vi "initialize_driver_session.vi"(4 "Supported instruments":string[](array[string]), 5 "Repeated Capabilities":T4[](array[typedef]), 6 "Attributes":T2[](array[typedef]) {"Flags" format="%08b"; "Access" items=["Read Only", "Write Only", "Read/Write"]; "Data Type" items=["Integer 32", "Double", "String", "Boolean", "None", "Integer 64", "RawString"]}, 7 "Range Tables":T3[](array[typedef]) {"Type" items=["Range", "Coerced", "Discrete"]}, 8 "error in":errorcluster caption="error in (no error)", 9 "Option String":string, 10 "Non-VXI sessions list (\"ASRL,SOCKET\")":T1[](array[typedef])=[enum."ASRL", enum."SOCKET"], 11 "VISA resource name":refnum<visa-resource-name>) -> (0 "error out":errorcluster, 2 "Simulation *IDN? response out":string, 3 "VISA resource name out":refnum<visa-resource-name>)   [LabVIEW 2020, in "Rohde&Schwarz RTx Oscilloscopes.lvlib" / "rsidr_core.lvlib"]
uses:
  rsidr_core.lvlib
  type_Input_Format_RepCap.ctl
  type_Input_Format_RangeTable.ctl
  type_Input_Format_Attribute.ctl
  type_InterfaceType.ctl
  type_Error_Codes.ctl
  type_Session_Parameter_int32.ctl
  type_Session_Data.ctl
  type_VisaAccessMode.ctl
  type_OPC_Wait_Mode.ctl
  type_Binary_Float_Number_Format.ctl
  type_Binary_Integer_Number_Format.ctl
  _type_Operation_Fgv_Attributes.ctl
  _type_Operation_Fgv_Cache.ctl
  _type_Operation_Fgv_RangeTable.ctl
  type_AdditionalFlag_Bits.ctl
  _type_Operation_Fgv_Session.ctl
  type_Session_Parameter_Boolean.ctl
  Match Regular Expression.xnode
  _type_Operation_Fgv_Debug.ctl
panel:
  # "Attribute Flags:\nbit 0: OPC Wait\nbit 1: No Status Check\nbit 2: Cache only\nbit 3: Hidden"
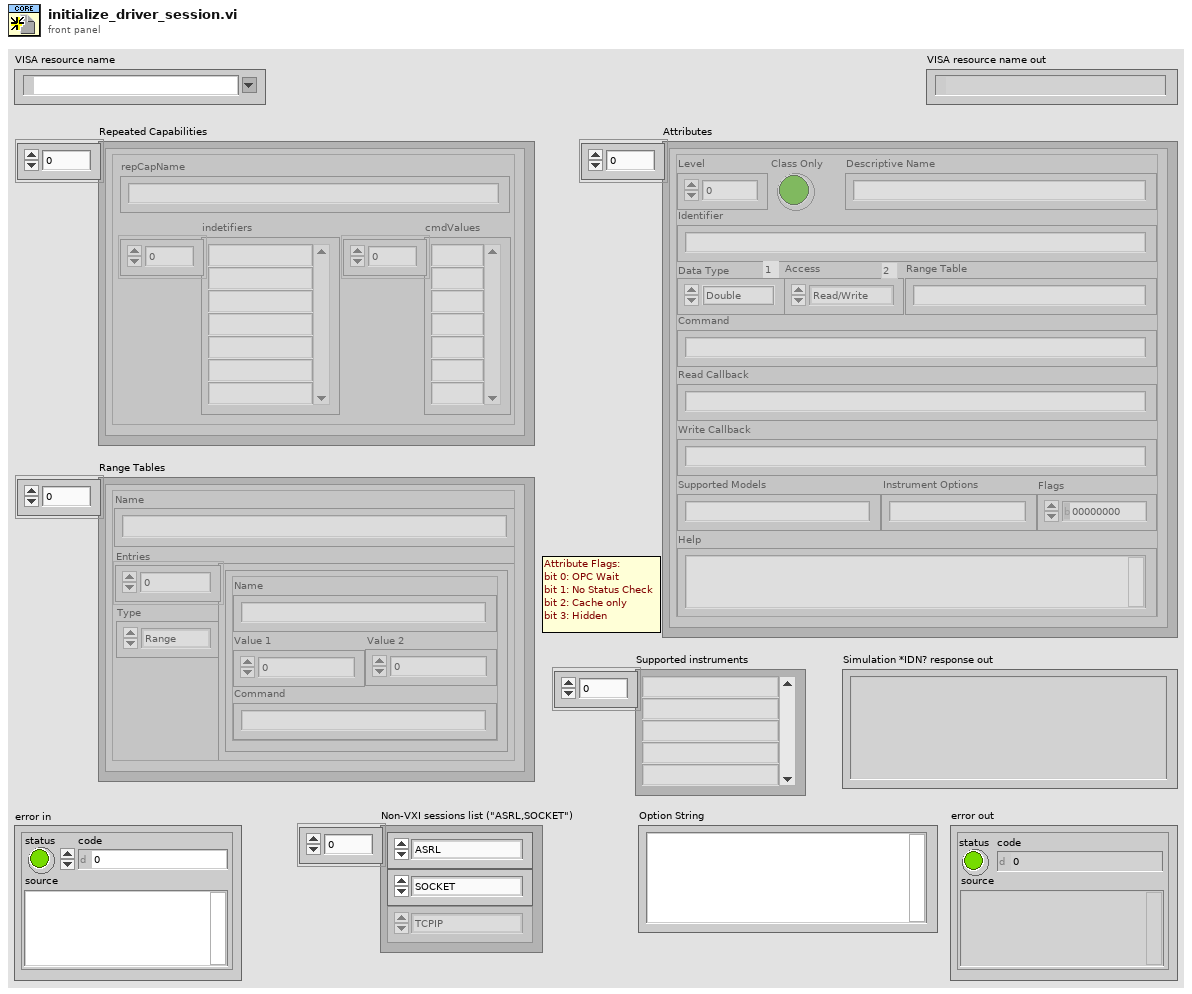
[diagram p1: front panel]
types:
  T1 = typedef "Rohde&Schwarz RTx Oscilloscopes.lvlib/rsidr_core.lvlib/type_InterfaceType.ctl" = enum16{"Unknown", "GPIB", "VXI", "GPIB_VXI", "ASRL", "PXI", "TCPIP", "USB", "SOCKET"}
  T2 = typedef "Rohde&Schwarz RTx Oscilloscopes.lvlib/rsidr_core.lvlib/type_Input_Format_Attribute.ctl" = cluster{"Level":i32, "Class Only":bool, "Identifier":string, "Descriptive Name":string, "Data Type":u16, "Command":string, "Access":u16, "Range Table":string, "Read Callback":string, "Write Callback":string, "Supported Models":string, "Instrument Options":string, "Flags":i32, "Help":string}
  T3 = typedef "Rohde&Schwarz RTx Oscilloscopes.lvlib/rsidr_core.lvlib/type_Input_Format_RangeTable.ctl" = cluster{"Type":u16, "Name":string, "Entries":cluster{"Name":string, "Value 1":dbl, "Value 2":dbl, "Command":string}[]}
  T4 = typedef "Rohde&Schwarz RTx Oscilloscopes.lvlib/rsidr_core.lvlib/type_Input_Format_RepCap.ctl" = cluster{"repCapName":string, "indetifiers":string[], "cmdValues":string[]}
  T5 = typedef "Rohde&Schwarz RTx Oscilloscopes.lvlib/rsidr_core.lvlib/_type_Operation_Fgv_RangeTable.ctl" = enum16{"Initialize", "Check", "Coerce", "Get Command String", "Get Numeric Value", "Get Default Value", "Get Range Table Type"}
  T6 = typedef "Rohde&Schwarz RTx Oscilloscopes.lvlib/rsidr_core.lvlib/_type_Operation_Fgv_Cache.ctl" = enum16{"Initialize", "Get Cached Value", "Set Cached Value", "Clear"}
  T7 = typedef "Rohde&Schwarz RTx Oscilloscopes.lvlib/rsidr_core.lvlib/_type_Operation_Fgv_Attributes.ctl" = enum16{"Initialize", "Get Attribute"}
  T8 = typedef "Rohde&Schwarz RTx Oscilloscopes.lvlib/rsidr_core.lvlib/type_Session_Data.ctl" = cluster{"IDN string":string, "Instrument FW":string, "Instr type":string, "Instr type for err. msg.":string, "Installed Options":string[], "Ignore Error Messages":string, "Logging params":variant, "OPC Timeout":i32, "VISA Timeout":i32, "STB Poll VISA Timeout":i32, "Additional Flags":i32, "Wait Before Read":i32, "Wait Before Write":i32, "Option String Flags":i32, "IO Segment Size":i64, "VISA Access Mode":T9, "Interface Type":T1, "OPC Wait Mode":T10, "Bin Float Number  Format":T11, "Bin Integer Number Format":T12, "Simulate":bool, "VXIcapable":bool, "Duplicate Session":bool, "Add LF to Write":bool, "Logging":bool, "Fast Sweep":bool, "Query Instrument Status":bool, "Check Range":bool, "Check Options":bool, "OPC-sync Attr Writes":bool, "OPC-sync Attr Queries":bool}
  T9 = typedef "Rohde&Schwarz RTx Oscilloscopes.lvlib/rsidr_core.lvlib/type_VisaAccessMode.ctl" = u16
  T10 = typedef "Rohde&Schwarz RTx Oscilloscopes.lvlib/rsidr_core.lvlib/type_OPC_Wait_Mode.ctl" = enum16{"STBpolling", "STBpollingSlow", "STBpollingSuperSlow", "ServiceRequest", "OPCquery"}
  T11 = typedef "Rohde&Schwarz RTx Oscilloscopes.lvlib/rsidr_core.lvlib/type_Binary_Float_Number_Format.ctl" = enum16{"Float_4_Bytes_Swapped", "Float_4_Bytes", "Double_8_Bytes_Swapped", "Double_8_Bytes"}
  T12 = typedef "Rohde&Schwarz RTx Oscilloscopes.lvlib/rsidr_core.lvlib/type_Binary_Integer_Number_Format.ctl" = enum16{"Int32_4_Bytes_Swapped", "Int32_4 Bytes", "Int16_2_Bytes_Swapped", "Int16_2_Bytes"}
  T13 = typedef "Rohde&Schwarz RTx Oscilloscopes.lvlib/rsidr_core.lvlib/type_Session_Parameter_int32.ctl" = enum16{"OPC Timeout", "Additional Flags", "Wait Before Write", "Wait Before Read", "Bin Data Chunk Size", "VISA Access Mode", "VISA Timeout", "Bin Float Number Format", "Bin Integer Number Format", "STBpollVISAtimeout", "OPCwaitMode"}
  T14 = typedef "Rohde&Schwarz RTx Oscilloscopes.lvlib/rsidr_core.lvlib/type_Error_Codes.ctl" = enum16{"No_error", "VISA_err_ResourceNotFound", "VISA_err_Timeout", "VISA_warn_MoreDataAvailable", "RS_err_MissingCallback", "RS_err_InvalidAttribute", "RS_err_InvalidValue", "RS_err_UnknownResource", "RS_err_AlreadyInitialized", "RS_err_InstrumentStatus", "RS_err_BadRepCapName", "RS_err_TypesMismatch", "RS_err_ValueNotSupported", "RS_err_InvalidRngTable", "RS_err_IDqueryFail", "RS_err_UnexpResponse", "VISA_warn_ConfigNotLoaded", "RS_err_AttributeNotReadable", "RS_err_AttributeNotWritable", "RS_err_InstrumentType", "RS_err_InstrumentOption", "VISA_err_InvalidSize", "RS_err_ReliabilityIndicator", "VISA_warn_UnknownStatus", "VISA_warn_TermCharRead", "VISA_err_IO_error", "RS_err_FunctionNotSupported", "VISA_warn_QueueEmpty"}
  T15 = typedef "Rohde&Schwarz RTx Oscilloscopes.lvlib/rsidr_core.lvlib/type_AdditionalFlag_Bits.ctl" = enum16{"Send LF after Bin Block", "Junk read with io_clear_buffers.vi", "io_clear_buffers: viClear()", "io_clear_buffers: viFlush()", "<NotUsed1>", "Allow Dbl & Int Bin/Ascii read", "*OPC? in check_instrument_error.vi", "<NotUsed2>", "Smart Enum Matching", "Less Strict RepCaps check", "AssureResponseEndWithLF"}
  T16 = typedef "Rohde&Schwarz RTx Oscilloscopes.lvlib/rsidr_core.lvlib/_type_Operation_Fgv_Session.ctl" = enum16{"Initialize", "GetData", "SetData", "Clear", "GetSessionIx"}
  T17 = typedef "Rohde&Schwarz RTx Oscilloscopes.lvlib/rsidr_core.lvlib/type_Session_Parameter_Boolean.ctl" = enum16{"Simulate", "Query Instr Status", "Check Range", "Check Options", "Add LF to Write", "Duplicate Session", "Fast Sweep", "Logging", "OPC-sync Attribute Queries", "OPC-sync Attribute Writes"}
  T18 = enum16{"Unknown", "GPIB", "VXI", "GPIB_VXI", "ASRL", "PXI", "TCPIP", "USB", "SOCKET"}
  T19 = typedef "Rohde&Schwarz RTx Oscilloscopes.lvlib/rsidr_core.lvlib/_type_Operation_Fgv_Debug.ctl" = enum16{"Reset", "ReadCommand", "SetCommand"}
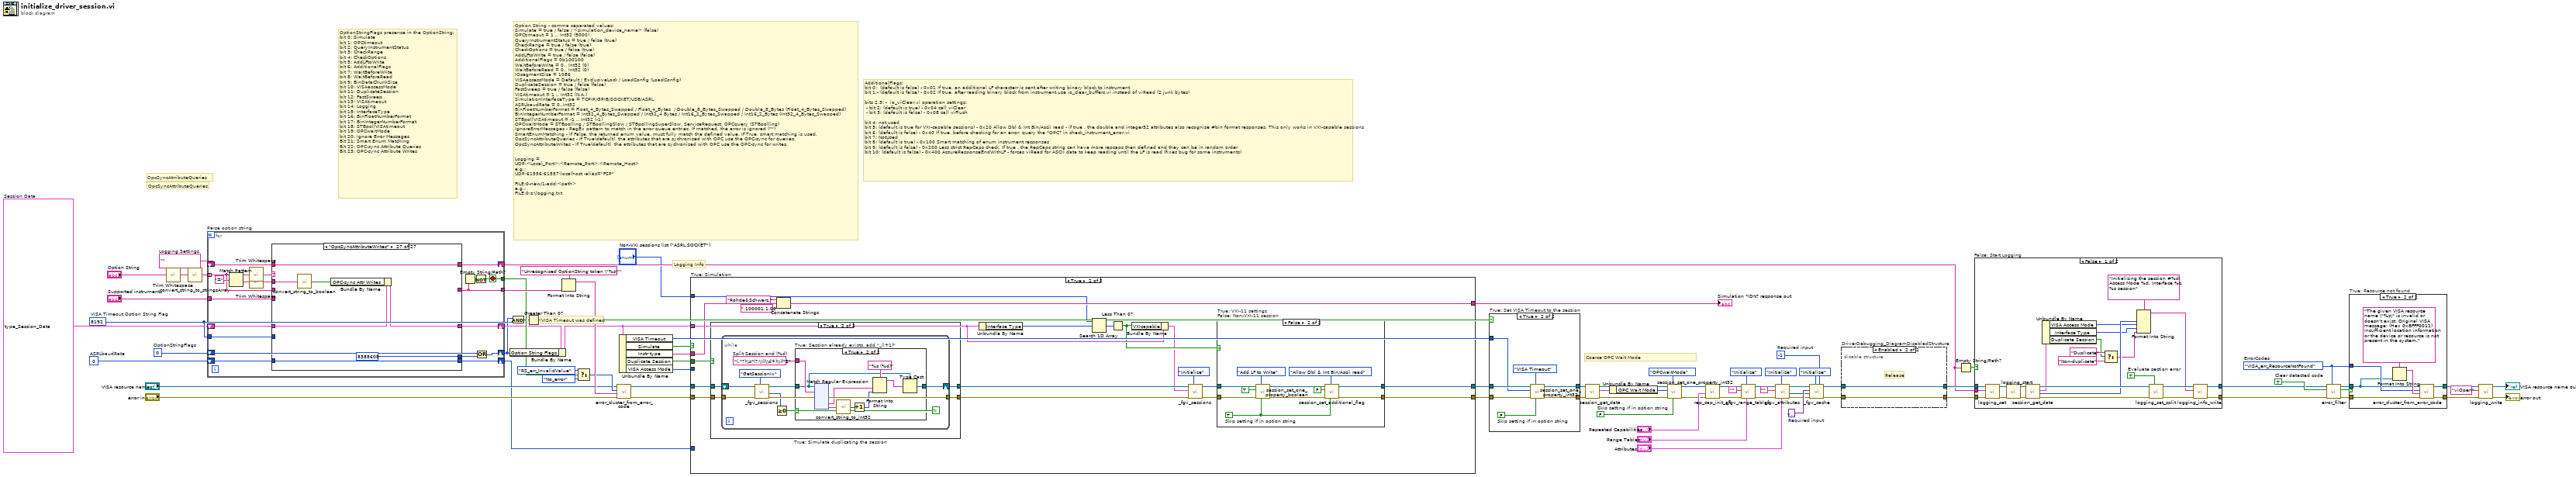
[diagram p0: block diagram]
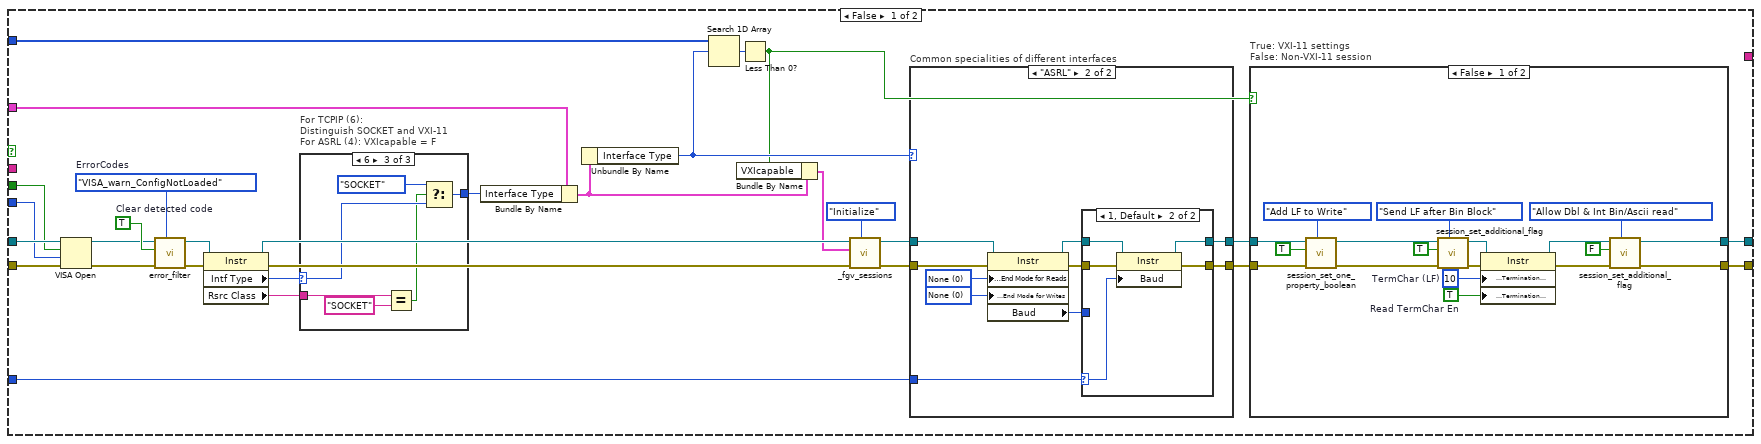
[diagram p3: hidden frame]
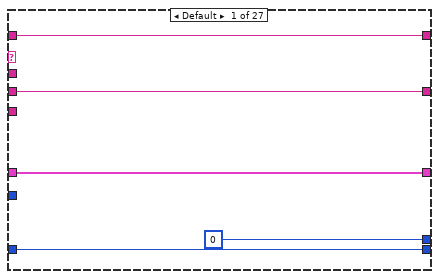
[diagram p14: hidden frame]
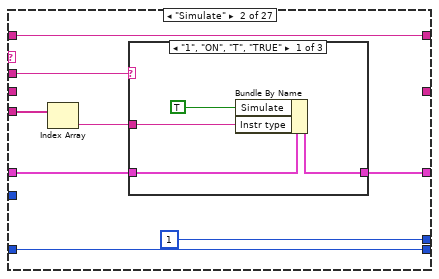
[diagram p15: hidden frame]
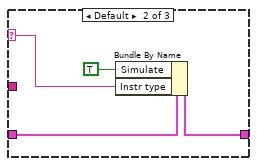
[diagram p16: hidden frame]
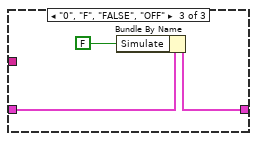
[diagram p17: hidden frame]
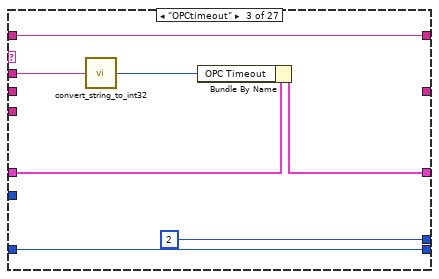
[diagram p18: hidden frame]
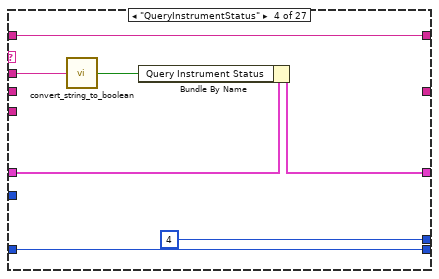
[diagram p19: hidden frame]
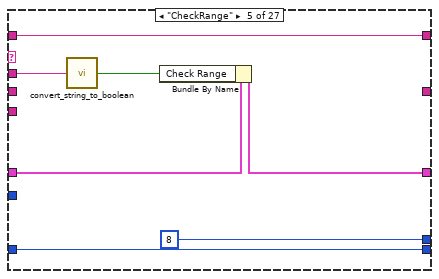
[diagram p20: hidden frame]
diagram:
  w4 = T8 {"IDN string"="", "Instrument FW"="", "Instr type"="", "Instr type for err. msg."="", "Installed Options"=[], "Ignore Error Messages"="", "Logging params"=variant, "OPC Timeout"=10000, "VISA Timeout"=5000, "STB Poll VISA Timeout"=-1, "Additional Flags"=292, "Wait Before Read"=0, "Wait Before Write"=0, "Option String Flags"=0, "IO Segment Size"=10000000, "VISA Access Mode"=4, "Interface Type"=enum."Unknown", "OPC Wait Mode"=enum."STBpolling", "Bin Float Number  Format"=enum."Float_4_Bytes_Swapped", "Bin Integer Number Format"=enum."Int32_4_Bytes_Swapped", "Simulate"=FALSE, "VXIcapable"=FALSE, "Duplicate Session"=FALSE, "Add LF to Write"=FALSE, "Logging"=FALSE, "Fast Sweep"=FALSE, "Query Instrument Status"=TRUE, "Check Range"=TRUE, "Check Options"=TRUE, "OPC-sync Attr Writes"=TRUE, "OPC-sync Attr Queries"=TRUE}  # Session Data
  w7 = FALSE  # Skip setting if in option string
  w18 = 0  # ASRLbaudRate
  w31 = 8192  # VISA Timeout Option String Flag
  w37 = 0  # OptionStringFlags
  w57 = type_Error_Codes."VISA_err_ResourceNotFound"  # ErrorCodes
  w59 = TRUE  # Clear detected code
  w66 = ""  # Logging Settings
  w80 = variant  # Required input
  w38 = -1  # Required input
  # "OpcSyncAttributeQueries"
  # "OpcSyncAtrributeQueries"
  # "Coerce OPC Wait Mode"
  # "VISA Timeout was defined"
  # "Logging Info"
  # "OptionStringFlags presence in the OptionString:\nbit 0: Simulate\nbit 1: OPCtimeout\nbit 2: QueryInstrumentStatus\nbit 3: CheckRange\nbit 4: CheckOptions\nbit 5: AddLFtoWrite\nbit 6: AdditionalFlags\nbit 7: WaitBeforeWrite\nbit 8: WaitBeforeRead\nbit 9: BinDataChunkSize\nbit 10: VISAaccessMode\nbit 11: DuplicateSession\nbit 12: FastSweep\nbit 13: VISAtimeout\nbit 14: Logging\nbit 15: InterfaceType\nbit 16: BinFloatNumberFormat\nbit 17: BinIntegerNumberFormat\nbit 18: STBpollVISAtimeout\nbit 19: OPCwaitMode\nbit 20: Ignore Error Messages\nBit 21: Smart Enum Matching\nBit 22: OPC-sync Attribute Queries\nBit 23: OPC-sync Attribute Writes"
  # "AdditionalFlags:\nbit 0:  (default is false) - 0x01 If true, an additional LF characterr is sent after writing binary block to instrument\nbit 1:- (default is false) - 0x02 If true, after reading binary block from instrument use io_clear_buffers.vi instead of viRead (2 junk bytes)\n\nbits 2,3: -  io_viClear.vi operation settings:\n - bit 2: (default is true) - 0x04 call viClear\n - bit 3: (default is false) - 0x08 call viFlush\n\nbit 4: not used\nbit 5: (default is true for VXI-capable sessions) - 0x20 Allow Dbl & Int Bin/Ascii read - if true , the double and integer32 attributes also recognise #bin format responses. This only works in VXI-capable sessions\nbit 6: (default is false) - 0x40 If true, before checking for an error, query the *OPC? in check_instrument_error.vi\nbit 7: NotUsed\nbit 8: (default is true) - 0x100 Smart matching of enum instrument responses\nbit 9: (default is false) - 0x200 Less strict RepCaps check. If true , the RepCaps string can have more repcaps then defined and they can be in random order\nbit 10: (default is false) - 0x400 AssureResponseEndWithLF - forces viRead for ASCII data to keep reading until the LF is read (fixes bug for some instruments)"
  # "Option String - comma separated values:\nSimulate = true / false / <simulation_device_name> (false)\nOPCtimeout = 1 .. Int32 (5000)\nQueryInstrumentStatus = true / false (true)\nCheckRange = true / false (true)\nCheckOptions = true / false (true)\nAddLFtoWrite = true / false (false)\nAdditionalFlags = 0b100100\nWaitBeforeWrite = 0.. Int32 (0)\nWaitBeforeRead = 0.. Int32 (0)\nIOsegmentSize = 10E6\nVISAaccessMode = Default / ExclusiveLock / LoadConfig (LoadConfig)\nDuplicateSession = true / false (false)\nFastSweep = true / false (false)\nVISAtimeout = 1 .. Int32 (N.A.)\nSimulationInterfaceType = TCPIP/GPIB/SOCKET/USB/ASRL\nASRLbaudRate = 0..Int32\nBinFloatNumberFormat = Float_4_Bytes_Swapped / Float_4_Bytes  / Double_8_Bytes_Swapped / Double_8_Bytes (Float_4_Bytes_Swapped)\nBinIntegerNumberFormat = Int32_4_Bytes_Swapped / Int32_4 Bytes / Int16_2_Bytes_Swapped / Int16_2_Bytes (Int32_4_Bytes_Swapped)\nSTBpollVISAtimeout = -1 .. Int32 (-1)\nOPCwaitMode = STBpolling / STBpollingSlow / STBpollingSuperSlow, ServiceRequest, OPCquery (STBpolling)\nIgnoreErrorMessages - RegEx pattern to match in the error queue entries. If matched, the error is ignored (\"\")\nSmartEnumMatching - If False, the returned enum value. must fully match the defined value. If True, smart matching is used.\nOpcSyncAttributeQueries - If True(default), the attributes that are sychronised with OPC use the OPC-sync for queries.\nOpcSyncAttributeWrites - If True(default), the attributes that are sychronised with OPC use the OPC-sync for writes.\n\n\nLogging =\nUDP:<Local_Port>:<Remote_Port>:<Remote_Host>\ne.g.:\nUDP:61556:61557:localhost -alias=\"FSP\"\n\nFILE:0-new/1-add:<path>\ne.g.:\nFILE:0:c:\\logging.txt"
  n1 = call "Trim Whitespace.vi"("string"="Option String") -> ("trimmed string"=w6:string)  [unwired: 1 in]
  n2 = call "convert_string_to_stringsArray.vi"("String in"=w6) -> ("string array out"=w70:string[])  [unwired: 3 in, 1 out]
  n3 = for "Parse option string" {
    tunnel: w70 -> [w94] mode=indexing
    shift-right: [w96] -> w33
    shift-left: w4 -> [w97]
    tunnel: "Supported instruments" -> [w92]
    shift-right: [w90] -> w64
    shift-left: w66 -> [w91]
    tunnel: [w88] -> w44
    tunnel: [w87] -> w43
    shift-right: [w85] -> w32
    shift-left: w37 -> [w86]
    tunnel: w31 -> [w83]
    shift-right: [w81] -> w17
    shift-left: w18 -> [w82]
    stop <- w87 stop-if-true
    n4 = Match Pattern(string=w94, regular expression="=") -> (before substring=w99:string, after substring=w98:string)  [unwired: 1 in, 2 out]
    n5 = call "Trim Whitespace.vi"("string"=w99) -> ("trimmed string"=w95:string)  [unwired: 1 in]
    n6 = call "Trim Whitespace.vi"("string"=w98) -> ("trimmed string"=w93:string)  [unwired: 1 in]
    n7 = case shown="\"OpcSyncAttributeWrites\"" w95 {
      tunnel: w97 -> [w105 w107 w131 w133 w140 w152 w154 w166 w173 w183 w190 w198 w200 w214 w221 w228 w235 w241 w244 w260 w275 w291 w297 w314 w324 w329 w336]
      tunnel: [w105 w106 w130 w132 w139 w146 w153 w165 w174 w182 w189 w197 w199 w213 w220 w227 w235 w241 w243 w259 w274 w290 w296 w313 w325 w328 w335] -> w96
      tunnel: w94 -> [w103 _ _ _ _ _ _ _ _ _ _ _ w205 _ _ _ _ _ w249 w265 w280 _ w302 _ _ _ _]
      tunnel: w93 -> [_ w109 w128 w137 w144 w150 w158 w163 w170 w180 w187 w195 w207 w218 w225 w232 w237 w242 w251 w267 w282 w293 w304 w312 w321 w333 w340]
      tunnel: w92 -> [_ w113 _ _ _ _ _ _ _ _ _ _ _ _ _ _ _ _ _ _ _ _ _ _ _ _ _]
      tunnel: w91 -> [w104 w112 w129 w138 w145 w151 w159 w164 w176 w181 w188 w196 w206 w219 w226 w233 w238 _ w250 w266 w281 w289 w303 w317 w327 w334 w341]
      tunnel: [w104 w112 w129 w138 w145 w151 w159 w164 w176 w181 w188 w196 w206 w219 w226 w233 w238 w242 w250 w266 w281 w289 w303 w317 w327 w334 w341] -> w90
      tunnel: [w103 _ _ _ _ _ _ _ _ _ _ _ w204 _ _ _ _ _ w248 w264 w279 _ w301 _ _ _ _] -> w88
      tunnel: [0 ("y") 1 ("y") 2 ("y") 4 ("y") 8 ("y") 16 ("y") 32 ("y") 64 ("y") 64 ("y") 128 ("y") 256 ("y") 512 ("y") 1024 ("y") 2048 ("y") 4096 ("y") w230 w234 16384 ("y") 32768 ("y") 65536 ("y") 131072 ("y") 262144 ("y") 524288 ("y") 1048576 ("y") 2097152 ("y") 4194304 ("y") 8388608 ("y")] -> w84
      tunnel: w83 -> [_ _ _ _ _ _ _ _ _ _ _ _ _ _ _ w230 _ _ _ _ _ _ _ _ _ _ _]
      tunnel: w82 -> [w101 w110 w125 w134 w141 w147 w155 w160 w175 w177 w184 w192 w201 w215 w222 w229 _ w239 w245 w261 w276 w294 w298 w315 w326 w330 w337]
      tunnel: [w101 w110 w125 w134 w141 w147 w155 w160 w175 w177 w184 w192 w201 w215 w222 w229 w236 w239 w245 w261 w276 w294 w298 w315 w326 w330 w337] -> w81
      frame Default {
      }
      frame "Simulate" {
        n8 = Index Array(array=w113) -> (element=w108:string)  [unwired: 1 in]
        n9 = case shown="\"1\", \"ON\", \"T\", \"TRUE\"" w109 {
          selector: w109 -> [_ w118 _]
          tunnel: w107 -> [w117 w121 w124]
          tunnel: [w116 w120 w123] -> w106
          tunnel: w108 -> [w115 _ _]
          frame "1", "ON", "T", "TRUE" {
            n10 = Bundle By Name(cluster=w117, "Simulate"=TRUE ("Simulation"), "Instr type"=w115) -> (w116:T8)
          }
          frame Default {
            n11 = Bundle By Name(cluster=w121, "Simulate"=TRUE ("Simulation"), "Instr type"=w118) -> (w120:T8)
          }
          frame "0", "F", "FALSE", "OFF" {
            n12 = Bundle By Name(cluster=w124, "Simulate"=FALSE ("Simulation")) -> (w123:T8)
          }
        }
      }
      frame "OPCtimeout" {
        n13 = call "convert_string_to_int32.vi"("String in"=w128) -> ("int32 value out"=w127:i32)  [unwired: 4 in]
        n14 = Bundle By Name(cluster=w131, "OPC Timeout"=w127) -> (w130:T8)
      }
      frame "QueryInstrumentStatus" {
        n15 = call "convert_string_to_boolean.vi"("String in"=w137) -> ("boolean value out"=w136:bool)  [unwired: 4 in]
        n16 = Bundle By Name(cluster=w133, "Query Instrument Status"=w136) -> (w132:T8)
      }
      frame "CheckRange" {
        n17 = call "convert_string_to_boolean.vi"("String in"=w144) -> ("boolean value out"=w143:bool)  [unwired: 4 in]
        n18 = Bundle By Name(cluster=w140, "Check Range"=w143) -> (w139:T8)
      }
      frame "CheckOptions" {
        n19 = call "convert_string_to_boolean.vi"("String in"=w150) -> ("boolean value out"=w149:bool)  [unwired: 4 in]
        n20 = Bundle By Name(cluster=w152, "Check Options"=w149) -> (w146:T8)
      }
      frame "AddLFtoWrite" {
        n21 = call "convert_string_to_boolean.vi"("String in"=w158) -> ("boolean value out"=w157:bool)  [unwired: 4 in]
        n22 = Bundle By Name(cluster=w154, "Add LF to Write"=w157) -> (w153:T8)
      }
      frame "AdditionalFlags" {
        n23 = call "convert_string_to_int32.vi"("String in"=w163) -> ("int32 value out"=w162:i32)  [unwired: 4 in]
        n24 = Bundle By Name(cluster=w166, "Additional Flags"=w162) -> (w165:T8)
      }
      frame "AssureResponseEndWithLF" {
        n25 = Unbundle By Name(w173) -> ("Additional Flags"=w172:i32)
        n26 = call "convert_string_to_boolean.vi"("String in"=w170) -> ("boolean value out"=w169:bool)  [unwired: 4 in]
        n27 = call "_session_set_additionalFlag_value.vi"("New value in"=w169, "AdditionalFlag bit"=type_AdditionalFlag_Bits."AssureResponseEndWithLF", "Additional Flags in"=w172) -> ("Additional Flags out"=w168:i32)  [unwired: 1 in, 1 out]
        n28 = Bundle By Name(cluster=w173, "Additional Flags"=w168) -> (w174:T8)
      }
      frame "WaitBeforeWrite" {
        n29 = call "convert_string_to_int32.vi"("String in"=w180) -> ("int32 value out"=w179:i32)  [unwired: 4 in]
        n30 = Bundle By Name(cluster=w183, "Wait Before Write"=w179) -> (w182:T8)
      }
      frame "WaitBeforeRead" {
        n31 = call "convert_string_to_int32.vi"("String in"=w187) -> ("int32 value out"=w186:i32)  [unwired: 4 in]
        n32 = Bundle By Name(cluster=w190, "Wait Before Read"=w186) -> (w189:T8)
      }
      frame "IOsegmentSize" {
        n33 = call "convert_string_to_int32.vi"("String in"=w195) -> ("int32 value out"=w194:i32)  [unwired: 4 in]
        n34 = To Quad Integer(1:w194) -> (0:w191:i64)
        n35 = Bundle By Name(cluster=w198, "IO Segment Size"=w191) -> (w197:T8)
      }
      frame "VISAaccessMode" {
        n36 = case shown="\"LoadConfig\"" w207 {
          tunnel: w205 -> [_ w210 _ _]
          tunnel: [_ w210 _ _] -> w204
          tunnel: [w208 w209 w211 w212] -> w203
          frame "Default" {
            w208 = T9 0 items=["VISA Defaults"=0, "Exclusive Lock"=1, "Load Settings"=4]  # VISA Access Mode
          }
          frame Default {
            w209 = T9 4 items=["VISA Defaults"=0, "Exclusive Lock"=1, "Load Settings"=4]  # VISA Access Mode
          }
          frame "ExclusiveLock" {
            w211 = T9 1 items=["VISA Defaults"=0, "Exclusive Lock"=1, "Load Settings"=4]  # VISA Access Mode
          }
          frame "LoadConfig" {
            w212 = T9 4 items=["VISA Defaults"=0, "Exclusive Lock"=1, "Load Settings"=4]  # VISA Access Mode
          }
        }
        n37 = Bundle By Name(cluster=w200, "VISA Access Mode"=w203) -> (w199:T8)
      }
      frame "DuplicateSession" {
        n38 = call "convert_string_to_boolean.vi"("String in"=w218) -> ("boolean value out"=w217:bool)  [unwired: 4 in]
        n39 = Bundle By Name(cluster=w214, "Duplicate Session"=w217) -> (w213:T8)
      }
      frame "FastSweep" {
        n40 = call "convert_string_to_boolean.vi"("String in"=w225) -> ("boolean value out"=w224:bool)  [unwired: 4 in]
        n41 = Bundle By Name(cluster=w221, "Fast Sweep"=w224) -> (w220:T8)
      }
      frame "VISAtimeout" {
        n42 = call "convert_string_to_int32.vi"("String in"=w232) -> ("int32 value out"=w231:i32)  [unwired: 4 in]
        n43 = Bundle By Name(cluster=w228, "VISA Timeout"=w231) -> (w227:T8)
      }
      frame "ASRLbaudRate" {
        w234 = 0  # OptionStringFlags
        n44 = call "convert_string_to_int32.vi"("String in"=w237) -> ("int32 value out"=w236:i32)  [unwired: 4 in]
      }
      frame "Logging" {
      }
      frame "SimulationInterfaceType" {
        n45 = case shown="\"ASRL\"" w251 {
          tunnel: w249 -> [w253 _ _ _ _ _]
          tunnel: [w253 _ _ _ _ _] -> w248
          tunnel: [type_InterfaceType."TCPIP" ("Interface Type") type_InterfaceType."TCPIP" ("Interface Type") type_InterfaceType."GPIB" ("Interface Type") type_InterfaceType."SOCKET" ("Interface Type") type_InterfaceType."USB" ("Interface Type") type_InterfaceType."ASRL" ("Interface Type")] -> w247
          frame Default {
          }
          frame "TCPIP" {
          }
          frame "GPIB" {
          }
          frame "SOCKET" {
          }
          frame "USB" {
          }
          frame "ASRL" {
          }
        }
        n46 = Bundle By Name(cluster=w244, "Interface Type"=w247) -> (w243:T8)
      }
      frame "BinFloatNumberFormat" {
        n47 = case shown="\"Double_8_Bytes_Swapped\"" w267 {
          tunnel: w265 -> [w269 _ _ _ _]
          tunnel: [w269 _ _ _ _] -> w264
          tunnel: [w268 w270 w271 w272 w273] -> w263
          frame Default {
            w268 = type_Binary_Float_Number_Format."Float_4_Bytes_Swapped"  # Bin Number Format
          }
          frame "Float_4_Bytes_Swapped" {
            w270 = type_Binary_Float_Number_Format."Float_4_Bytes_Swapped"  # Bin Float Number Format
          }
          frame "Float_4_Bytes" {
            w271 = type_Binary_Float_Number_Format."Float_4_Bytes"  # Bin Float Number Format
          }
          frame "Double_8_Bytes_Swapped" {
            w272 = type_Binary_Float_Number_Format."Double_8_Bytes_Swapped"  # Bin Float Number Format
          }
          frame "Double_8_Bytes" {
            w273 = type_Binary_Float_Number_Format."Double_8_Bytes"  # Bin Float Number Format
          }
        }
        n48 = Bundle By Name(cluster=w260, "Bin Float Number  Format"=w263) -> (w259:T8)
      }
      frame "BinIntegerNumberFormat" {
        n49 = case shown="\"Int16_2_Bytes_Swapped\"" w282 {
          tunnel: w280 -> [w284 _ _ _ _]
          tunnel: [w284 _ _ _ _] -> w279
          tunnel: [w283 w285 w286 w287 w288] -> w278
          frame Default {
            w283 = type_Binary_Integer_Number_Format."Int32_4_Bytes_Swapped"  # Bin Integer Number Format
          }
          frame "Int32_4_Bytes_Swapped" {
            w285 = type_Binary_Integer_Number_Format."Int32_4_Bytes_Swapped"  # Bin Integer Number Format
          }
          frame "Int32_4_Bytes" {
            w286 = type_Binary_Integer_Number_Format."Int32_4 Bytes"  # Bin Integer Number Format
          }
          frame "Int16_2_Bytes_Swapped" {
            w287 = type_Binary_Integer_Number_Format."Int16_2_Bytes_Swapped"  # Bin Integer Number Format
          }
          frame "Int16_2_Bytes" {
            w288 = type_Binary_Integer_Number_Format."Int16_2_Bytes"  # Bin Integer Number Format
          }
        }
        n50 = Bundle By Name(cluster=w275, "Bin Integer Number Format"=w278) -> (w274:T8)
      }
      frame "STBpollVISAtimeout" {
        n51 = call "convert_string_to_int32.vi"("String in"=w293) -> ("int32 value out"=w292:i32)  [unwired: 4 in]
        n52 = Bundle By Name(cluster=w291, "STB Poll VISA Timeout"=w292) -> (w290:T8)
      }
      frame "OPCwaitMode" {
        n53 = case shown="Default" w304 {
          tunnel: w302 -> [_ _ _ _ _ w310]
          tunnel: [_ _ _ _ _ w310] -> w301
          tunnel: [w305 w306 w307 w308 w309 w311] -> w300
          frame "STBpolling" {
            w305 = type_OPC_Wait_Mode."STBpolling"  # OPC Wait Mode
          }
          frame "STBpollingSlow" {
            w306 = type_OPC_Wait_Mode."STBpollingSlow"  # OPC Wait Mode
          }
          frame "STBpollingSuperSlow" {
            w307 = type_OPC_Wait_Mode."STBpollingSuperSlow"  # OPC Wait Mode
          }
          frame "ServiceRequest" {
            w308 = type_OPC_Wait_Mode."ServiceRequest"  # OPC Wait Mode
          }
          frame "OPCquery" {
            w309 = type_OPC_Wait_Mode."OPCquery"  # OPC Wait Mode
          }
          frame Default {
            w311 = type_OPC_Wait_Mode."STBpolling"  # OPC Wait Mode
          }
        }
        n54 = Bundle By Name(cluster=w297, "OPC Wait Mode"=w300) -> (w296:T8)
      }
      frame "IgnoreErrorMessages" {
        n55 = Bundle By Name(cluster=w314, "Ignore Error Messages"=w312) -> (w313:T8)
      }
      frame "SmartEnumMatching" {
        n56 = Unbundle By Name(w324) -> ("Additional Flags"=w323:i32)
        n57 = call "convert_string_to_boolean.vi"("String in"=w321) -> ("boolean value out"=w320:bool)  [unwired: 4 in]
        n58 = call "_session_set_additionalFlag_value.vi"("New value in"=w320, "AdditionalFlag bit"=type_AdditionalFlag_Bits."Smart Enum Matching", "Additional Flags in"=w323) -> ("Additional Flags out"=w319:i32)  [unwired: 1 in, 1 out]
        n59 = Bundle By Name(cluster=w324, "Additional Flags"=w319) -> (w325:T8)
      }
      frame "OpcSyncAttributeQueries" {
        n60 = call "convert_string_to_boolean.vi"("String in"=w333) -> ("boolean value out"=w332:bool)  [unwired: 4 in]
        n61 = Bundle By Name(cluster=w329, "OPC-sync Attr Queries"=w332) -> (w328:T8)
      }
      frame "OpcSyncAttributeWrites" {
        n62 = call "convert_string_to_boolean.vi"("String in"=w340) -> ("boolean value out"=w339:bool)  [unwired: 4 in]
        n63 = Bundle By Name(cluster=w336, "OPC-sync Attr Writes"=w339) -> (w335:T8)
      }
    }
    n64 = Empty String/Path?(string/path=w88) -> (empty?=w89:bool)
    n65 = Not(x=w89) -> (.not. x?=w87:bool)
    n66 = Or(x=w86, y=w84) -> (x .or. y?=w85:i32)
  }
  n67 = Bundle By Name(cluster=w33, "Option String Flags"=w32) -> (w36:T8)
  n68 = And(x=w32, y=w31) -> (x .and. y?=w30:i32)
  n69 = Greater Than 0?(x=w30) -> (x > 0?=w29:bool)
  n70 = Format Into String(format string="Unrecognised OptionString token \"%s\"", w44) -> (resulting string=w46:string)  [unwired: 2 in, 1 out]
  n71 = Select(t=type_Error_Codes."RS_err_InvalidValue" ("Error Enum in"), s=w43, f=type_Error_Codes."No_error" ("Error Enum in")) -> (s? t:f=w40:T14)
  n72 = call "error_cluster_from_error_code.vi"("error in"="error in", "Error Message (\"\")"=w46, "Error Enum in"=w40, "VISA resource name"="VISA resource name") -> ("error out"=w25:errorcluster, "VISA resource name out"=w24:refnum<visa-resource-name>)  [unwired: 6 in]
  n73 = Unbundle By Name(w36) -> ("VISA Timeout"=w28:i32, "Simulate"=w56:bool, "Instr type"=w58:string, "Duplicate Session"=w23:bool, "VISA Access Mode"=w22:T9)
  n74 = case "True: Simulation" shown="True" w56 {
    tunnel: w24 -> [w370 w435]
    tunnel: w25 -> [w371 w434]
    tunnel: [w350 w428] -> w35
    tunnel: [w349 w427] -> w34
    tunnel: w58 -> [_ w433]
    tunnel: [_ w437] -> w55
    tunnel: w36 -> [w360 w426]
    tunnel: w23 -> [w363 w436]
    tunnel: w22 -> [w362 _]
    tunnel: w17 -> [w353 _]
    tunnel: "Non-VXI sessions list (\"ASRL,SOCKET\")" -> [w347 w424]
    frame False {
      w364 = TRUE  # Clear detected code
      w367 = type_Error_Codes."VISA_warn_ConfigNotLoaded"  # ErrorCodes
      n75 = VISA Open ("Open instrument")(duplicate session (F)=w363, access mode=w362, error in (no error)=w371, VISA resource name=w370) -> (VISA resource name=w359:refnum<visa-resource-name>, error out=w358:errorcluster)  [unwired: 1 in]
      n76 = call "error_filter.vi"("Error Enum in"=w367, "error in"=w358, "Clear detected code (F)"=w364, "VISA resource name"=w359) -> ("error out"=w366:errorcluster, "VISA resource name out"=w365:refnum<visa-resource-name>)  [unwired: 5 in, 1 out]
      n77 = property on="Property Node" class="Instr"(reference=w365, error in=w366) -> (reference out=w356:refnum<visa-resource-name>, error out=w357:errorcluster, "Intf Type"=w369:u16, "Rsrc Class"=w368:string)
      n78 = case "For TCPIP (6):\nDistinguish SOCKET and VXI-11\nFor ASRL (4): VXIcapable = F" shown="6" w369 {
        selector: w369 -> [w411 w412 w416]
        tunnel: w368 -> [_ _ w418]
        tunnel: [w411 w412 w415] -> w361
        frame Default {
        }
        frame 4 {
        }
        frame 6 {
          n79 = Equal?(x=w418, y="SOCKET") -> (x = y?=w413:bool)
          n80 = Select(t=T18."SOCKET" ("Interface Type"), s=w413, f=w416) -> (s? t:f=w415:u16)
        }
      }
      n81 = Bundle By Name(cluster=w360, "Interface Type"=w361) -> (w344:T8)
      n82 = Unbundle By Name(w344) -> ("Interface Type"=w346:T1)
      n83 = Search 1D Array(1D array=w347, element=w346) -> (index of element=w348:i32)  [unwired: 1 in]
      n84 = Less Than 0?(x=w348) -> (x < 0?=w343:bool)
      n85 = Bundle By Name(cluster=w344, "VXIcapable"=w343) -> (w345:T8)
      n86 = call "_fgv_sessions.vi"("Operation"=_type_Operation_Fgv_Session."Initialize", "error in"=w357, "Session User Data in (None)"=w345, "VISA resource name"=w356) -> ("error out"=w355:errorcluster, "VISA resource name out"=w354:refnum<visa-resource-name>)  [unwired: 4 in, 2 out]
      n87 = case "Common specialities of different interfaces" shown="\"ASRL\"" w346 {
        tunnel: w355 -> [w392 w396]
        tunnel: w354 -> [w393 w395]
        tunnel: [w392 w398] -> w352
        tunnel: [w393 w397] -> w351
        tunnel: w353 -> [_ w401]
        frame Default {
        }
        frame "ASRL" {
          w402 = u16 0 items=["None", "Last Bit", "TermChar", "Break"] ("Serial Settings:End Mode for Writes")
          w403 = u16 0 items=["None", "Last Bit", "TermChar"] ("Serial Settings:End Mode for Reads")
          n88 = property on="Property Node" class="Instr"(reference=w395, error in=w396, "Serial Settings:End Mode for Reads"=w403, "Serial Settings:End Mode for Writes"=w402) -> (reference out=w399:refnum<visa-resource-name>, error out=w400:errorcluster, "Baud"=w394:u32)
          n89 = case shown="1, Default" w401 {
            selector: w401 -> [_ w406]
            tunnel: w400 -> [w404 w410]
            tunnel: w399 -> [w405 w407]
            tunnel: [w404 w409] -> w398
            tunnel: [w405 w408] -> w397
            tunnel: w394 -> [_ _]
            frame 0 {
            }
            frame 1, Default {
              n90 = property on="Property Node" class="Instr"(reference=w407, error in=w410, "Baud"=w406) -> (reference out=w408:refnum<visa-resource-name>, error out=w409:errorcluster)
            }
          }
        }
      }
      n91 = case "True: VXI-11 settings\nFalse: Non-VXI-11 session" shown="False" w343 {
        tunnel: w352 -> [w386 w390]
        tunnel: w351 -> [w387 w391]
        tunnel: [w375 w390] -> w350
        tunnel: [w374 w391] -> w349
        frame False {
          w388 = u8 10  # TermChar (LF)
          w389 = TRUE  # Read TermChar En
          n92 = call "session_set_one_property_boolean.vi"("Session Parameter Boolean"=type_Session_Parameter_Boolean."Add LF to Write" ("Session Parameter boolean"), "error in"=w386, "Boolean value in"=TRUE ("boolean value in"), "VISA resource name"=w387) -> ("error out"=w383:errorcluster, "VISA resource name out"=w384:refnum<visa-resource-name>)  [unwired: 5 in, 1 out]
          n93 = call "session_set_additional_flag.vi"("AdditionalFlag Bit"=type_AdditionalFlag_Bits."Send LF after Bin Block" ("AdditionalFlag bit"), "error in"=w383, "New value in"=TRUE, "VISA resource name"=w384) -> ("error out"=w381:errorcluster, "VISA resource name out"=w382:refnum<visa-resource-name>)  [unwired: 5 in, 1 out]
          n94 = property on="Property Node" class="Instr"(reference=w382, error in=w381, "Message Based Settings:Termination Character"=w388, "Message Based Settings:Termination Character Enable"=w389) -> (reference out=w373:refnum<visa-resource-name>, error out=w376:errorcluster)
          n95 = call "session_set_additional_flag.vi"("AdditionalFlag Bit"=type_AdditionalFlag_Bits."Allow Dbl & Int Bin/Ascii read" ("AdditionalFlag bit"), "error in"=w376, "New value in"=FALSE, "VISA resource name"=w373) -> ("error out"=w375:errorcluster, "VISA resource name out"=w374:refnum<visa-resource-name>)  [unwired: 5 in, 1 out]
        }
        frame True {
        }
      }
    }
    frame True {
      n96 = case "True: Simulate duplicating the session" shown="True" w436 {
        tunnel: w435 -> [w453 w455]
        tunnel: [w453 w454] -> w431
        tunnel: w434 -> [w452 w457]
        tunnel: [w452 w456] -> w432
        frame False {
        }
        frame True {
          n97 = while {
            tunnel: w457 -> [w466]
            tunnel: [w465] -> w456
            shift-right: [w460] -> w454
            shift-left: w455 -> [w464]
            stop <- w459 continue-if-true
            w461 = "(.*?)\\s*(?:\\((\\d+)\\))*$"  # Split Session and (%d)
            n98 = call "_fgv_sessions.vi"("Operation"=_type_Operation_Fgv_Session."GetSessionIx", "error in"=w466, "VISA resource name"=w464) -> ("error out"=w465:errorcluster, "Session Ix out"=w463:i32, "VISA resource name out"=w462:refnum<visa-resource-name>)  [unwired: 5 in, 1 out]
            n99 = Greater Or Equal To 0?(x=w463) -> (x >= 0?=w459:bool)
            n100 = case "True: Session already exists, add \"_(i+1)\"" shown="True" w459 {
              tunnel: w462 -> [w467 w468]
              tunnel: w461 -> [_ w476]
              tunnel: [w467 w469] -> w460
              frame False {
              }
              frame True {
                n101 = xnode "Match Regular Expression"("input string"=w468, "regular expression"=w476) -> ("submatch 1"=w472:string, "submatch 2"=w475:string)  [unwired: 4 in, 5 out]
                n102 = call "convert_string_to_int32.vi"("String in"=w475) -> ("int32 value out"=w474:i32)  [unwired: 4 in]
                n103 = Increment(x=w474) -> (x+1=w471:i32)
                n104 = Format Into String(format string="%s (%d)", w472, w471) -> (resulting string=w470:string)  [unwired: 2 in, 1 out]
                n105 = Type Cast(type=w468, x=w470) -> (*(type *) &x=w469:refnum<visa-resource-name>)
              }
            }
          }
        }
      }
      n106 = Concatenate Strings("Rohde&Schwarz," ("read buffer"), w433, ",100001,1.00" ("string")) -> (w437:string)
      n107 = Unbundle By Name(w426) -> ("Interface Type"=w425:T1)
      n108 = Search 1D Array(1D array=w424, element=w425) -> (index of element=w423:i32)  [unwired: 1 in]
      n109 = Less Than 0?(x=w423) -> (x < 0?=w422:bool)
      n110 = Bundle By Name(cluster=w426, "VXIcapable"=w422) -> (w421:T8)
      n111 = call "_fgv_sessions.vi"("Operation"=_type_Operation_Fgv_Session."Initialize", "error in"=w432, "Session User Data in (None)"=w421, "VISA resource name"=w431) -> ("error out"=w430:errorcluster, "VISA resource name out"=w429:refnum<visa-resource-name>)  [unwired: 4 in, 2 out]
      n112 = case "True: VXI-11 settings\nFalse: Non-VXI-11 session" shown="False" w422 {
        tunnel: w430 -> [w439 w450]
        tunnel: w429 -> [w440 w449]
        tunnel: [w439 w445] -> w428
        tunnel: [w440 w444] -> w427
        frame True {
        }
        frame False {
          w441 = TRUE  # Skip setting if in option string
          n113 = call "session_set_one_property_boolean.vi"("Skip setting if in Options string (F)"=w441, "Session Parameter Boolean"=type_Session_Parameter_Boolean."Add LF to Write" ("Session Parameter boolean"), "error in"=w450, "Boolean value in"=TRUE ("boolean value in"), "VISA resource name"=w449) -> ("error out"=w447:errorcluster, "VISA resource name out"=w446:refnum<visa-resource-name>)  [unwired: 4 in, 1 out]
          n114 = call "session_set_additional_flag.vi"("Skip setting if in Options string (F)"=w441, "AdditionalFlag Bit"=type_AdditionalFlag_Bits."Allow Dbl & Int Bin/Ascii read" ("AdditionalFlag bit"), "error in"=w447, "New value in"=FALSE, "VISA resource name"=w446) -> ("error out"=w445:errorcluster, "VISA resource name out"=w444:refnum<visa-resource-name>)  [unwired: 4 in, 1 out]
        }
      }
    }
  }
  "Simulation *IDN? response out" <- w55
  n115 = case "True: Set VISA Timeout to the session" shown="True" w29 {
    tunnel: w35 -> [w591 w599]
    tunnel: w34 -> [w592 w598]
    tunnel: [w591 w597] -> w13
    tunnel: [w592 w596] -> w12
    tunnel: w28 -> [_ w595]
    frame False {
    }
    frame True {
      w593 = FALSE  # Skip setting if in option string
      n116 = call "session_set_one_property_int32.vi"("Skip setting if in Options string (F)"=w593, "Session Parameter Integer"=type_Session_Parameter_int32."VISA Timeout" ("Session Parameter to set"), "error in"=w599, "Int32 value in"=w595, "VISA resource name"=w598) -> ("error out"=w597:errorcluster, "VISA resource name out"=w596:refnum<visa-resource-name>)  [unwired: 4 in, 1 out]
    }
  }
  n117 = call "session_get_data.vi"("error in"=w13, "VISA resource name"=w12) -> ("error out"=w11:errorcluster, "Session User Data out"=w9:T8, "VISA resource name out"=w10:refnum<visa-resource-name>)  [unwired: 6 in, 1 out]
  n118 = Unbundle By Name(w9) -> ("OPC Wait Mode"=w8:T10)
  n119 = call "session_set_one_property_int32.vi"("Skip setting if in Options string (F)"=w7, "Session Parameter Integer"=type_Session_Parameter_int32."OPCwaitMode" ("Session Parameter to set"), "error in"=w11, "Int32 value in"=w8, "VISA resource name"=w10) -> ("error out"=w15:errorcluster, "VISA resource name out"=w14:refnum<visa-resource-name>)  [unwired: 4 in, 1 out]
  n120 = call "rep_cap_init_all.vi"("error in"=w15, "Repeated Capabilities"="Repeated Capabilities", "VISA resource name"=w14) -> ("error out"=w63:errorcluster, "VISA resource name out"=w21:refnum<visa-resource-name>)  [unwired: 7 in]
  n121 = call "_fgv_range_tables.vi"("Range Tables (empty)"="Range Tables", "Operation"=_type_Operation_Fgv_RangeTable."Initialize", "error in"=w63, "Range Table ID in"="" ("Empty String Constant"), "VISA resource name"=w21) -> ("error out"=w77:errorcluster, "VISA resource name out"=w19:refnum<visa-resource-name>)  [unwired: 2 in, 3 out]
  n122 = call "_fgv_attributes.vi"("Attributes (empty)"="Attributes", "Operation"=_type_Operation_Fgv_Attributes."Initialize", "error in"=w77, "Attribute ID in"="" ("Empty String Constant"), "VISA resource name"=w19) -> ("error out"=w76:errorcluster, "Count Out"=w39:i32, "VISA resource name out"=w20:refnum<visa-resource-name>)  [unwired: 3 in, 1 out]
  n123 = call "_fgv_cache.vi"("Index in"=w38, "Operation"=_type_Operation_Fgv_Cache."Initialize", "error in"=w76, "Initialization Count (0)"=w39, "Value in"=w80, "VISA resource name"=w20) -> ("error out"=w73:errorcluster, "VISA resource name out"=w72:refnum<visa-resource-name>)  [unwired: 3 in, 1 out]
  n124 = disable-structure "DriverDebugging_DiagramDisabledStructure" shown="Enabled" {
    disable-tunnel: w73 -> [w605 w606]
    disable-tunnel: [w603 w606] -> w68
    disable-tunnel: w72 -> [w604 w607]
    disable-tunnel: [w602 w607] -> w67
    frame Disabled {
      # "Debug"
      n125 = call "_fgv_debug.vi"("Operation"=_type_Operation_Fgv_Debug."Reset", "error in"=w605, "Command in"="" ("Empty String Constant"), "VISA resource name"=w604) -> ("error out"=w603:errorcluster, "VISA resource name out"=w602:refnum<visa-resource-name>)  [unwired: 6 in]
    }
    frame Enabled {
      # "Release"
    }
  }
  n126 = Empty String/Path?(string/path=w64) -> (empty?=w65:bool)
  n127 = case "False: Start Logging" shown="False" w65 {
    tunnel: w68 -> [w630 w632]
    tunnel: w67 -> [w629 w633]
    tunnel: [w624 w632] -> w47
    tunnel: [w623 w633] -> w48
    tunnel: w64 -> [w631 _]
    frame False {
      w609 = TRUE  # Evaluate section error
      n128 = call "logging_set.vi"("error in"=w630, "Logging target"=w631, "VISA resource name"=w629) -> ("error out"=w628:errorcluster, "VISA resource name out"=w627:refnum<visa-resource-name>)  [unwired: 7 in]
      n129 = call "logging_start.vi"("error in"=w628, "VISA resource name"=w627) -> ("error out"=w622:errorcluster, "VISA resource name out"=w621:refnum<visa-resource-name>)  [unwired: 8 in]
      n130 = call "session_get_data.vi"("error in"=w622, "VISA resource name"=w621) -> ("error out"=w620:errorcluster, "Session Ix out"=w614:i32, "Session User Data out"=w618:T8, "VISA resource name out"=w619:refnum<visa-resource-name>)  [unwired: 6 in]
      n131 = Unbundle By Name(w618) -> ("VISA Access Mode"=w613:T9, "Interface Type"=w612:T1, "Duplicate Session"=w608:bool)
      n132 = Select(t="Duplicate", s=w608, f="Non-duplicate") -> (s? t:f=w611:string)
      n133 = Format Into String(format string="Initializing the session #%d: Access Mode %d, Interface %s, %s session", w614, w613, w612, w611) -> (resulting string=w610:string)  [unwired: 2 in, 1 out]
      n134 = call "logging_set_split.vi"("Evaluate section error (F)"=w609, "error in"=w620, "VISA resource name"=w619) -> ("error out"=w626:errorcluster, "VISA resource name out"=w625:refnum<visa-resource-name>)  [unwired: 7 in]
      n135 = call "logging_info_write.vi"("error in"=w626, "String to write"=w610, "VISA resource name"=w625) -> ("error out"=w624:errorcluster, "VISA resource name out"=w623:refnum<visa-resource-name>)  [unwired: 7 in]
    }
    frame True {
    }
  }
  n136 = call "error_filter.vi"("Error Enum in"=w57, "error in"=w47, "Clear detected code (F)"=w59, "VISA resource name"=w48) -> ("error out"=w60:errorcluster, "Code Detected"=w61:bool, "VISA resource name out"=w49:refnum<visa-resource-name>)  [unwired: 5 in]
  n137 = case "True: Resource not found" shown="True" w61 {
    tunnel: w60 -> [w635 w640]
    tunnel: [w635 w642] -> w53
    tunnel: w49 -> [w634 w636]
    tunnel: w57 -> [_ w638]
    tunnel: [w634 w637] -> w52
    frame False {
    }
    frame True {
      n138 = Format Into String(format string="The given VISA resource name \"%s\" is invalid or doesn't exist. Original VISA message: (Hex 0xBFFF0011) Insufficient location information or the device or resource is not present in the system.", w636) -> (resulting string=w639:string)  [unwired: 2 in, 1 out]
      n139 = call "error_cluster_from_error_code.vi"("error in"=w640, "Error Message (\"\")"=w639, "Error Enum in"=w638, "VISA resource name"=w636) -> ("error out"=w642:errorcluster, "VISA resource name out"=w637:refnum<visa-resource-name>)  [unwired: 6 in]
    }
  }
  n140 = call "logging_write.vi"("error in"=w53, "String to write"="viOpen", "VISA resource name"=w52) -> ("error out"=→"error out":errorcluster, "VISA resource name out"=→"VISA resource name out":refnum<visa-resource-name>)  [unwired: 7 in]
